vi "CAN Position Control Encoder.vi"() -> ()   [LabVIEW 2014]
doc: "This example shows how to position a motor using CAN Jaguar and a quadrature encoder. For details setting up and understanding CAN Jaguar, see the Can Jaguar Fundamentals tutorial accessable from the LabVIEW Getting Started Window.\n\nTo position the motor, a PID control loop runs on the Jaguar. Notice that the encoder is wired directly to the Jaguar. One advantage of this is that the PID control does not use resources on the roboRIO. One disadvantage is that the PID code cannot be viewed or changed. However, the control can be tuned by changing the PID Parameters.\n\nOn the diagram, notice that in order to apply new PID tuning parameters, the motor must first be disabled, and then enabled afterward. Also notice that since the control loop runs on the Jaguar, the LabVIEW loop delay is set to a slow 100ms. In fact the only reason this loop needs to run is to send a new set position, read the current position, or apply new tuning parameters.\n\nCorrect tuning parameters for a PID controller are dependent on the complete system of the motor and the load. It will be difficult to tune this system if there is no load attached to the motor. While this example is not a PID tutorial, the following information may help in understanding how to tune your PID control system.\n\nP (proportional) depends on the present error, I (integral) on the accumulation of past errors, and D (derivative) is a prediction of future errors, based on the current rate of change. The proportional parameter (P) will reduce the rise time and will reduce, but never eliminate, the steady-state error. The integral parameter (I) will eliminate the steady-state error, but may make the transient response worse. The derivative parameter (D) will increase the stability of the system, reducing the overshoot, and improving the transient response. The effects of each parameter are summarized in a table on the front panel.\n\nThis example expects a USB cable connected from your development PC to the Type B USB Jack (next to the power input) on the roboRIO.\n\nThis example requires the Driver Station to be running with Teleoperated Enabled."
uses:
  <vilib>/Rock Robotics/WPI/CAN/Jaguar/SubVIs/WPI_CANJaguar_PositionReference.ctl
  <vilib>/Rock Robotics/WPI/CAN/TalonSRX/WPI_CANTalonSRX_APIControlMode.ctl
  <vilib>/Rock Robotics/WPI/MotorControl/WPI_MotorControlOpenCANTalonSRX.vi
panel:
  in  "PID Tuning":string[][](table)=[["Parameter", "Rise Time", "Overshoot", "Settling\nTime", "Steady State\nError"], ["P", "decrease", "increase", "small\nchange", "decrease"], ["I", "decrease", "increase", "increase", "eliminate"], ["D", "small\nchange", "decrease", "decrease", "small\nchange"]]
  out "Actual Position (revolutions)":dbl(slide) scale=-10.0..10.0
  in  "D2":dbl=15.0 caption="D"
  in  "I2":dbl=0.005 caption="I"
  in  "P2":dbl=500.0 caption="P"
  in  "apply new PID":bool
  in  "D":dbl=15.0
  in  "I":dbl=0.005
  in  "P":dbl=500.0
  in  "Set Position (revolutions)":dbl(slide) scale=-10.0..10.0
  in  "Device Number":u8=1
  in  "stop":bool
  # "Set these inputs before running."
  # "These can be set while running."
  # "Power\nTerminals"
  # "Motor\nTerminals"
  # "Looking at the RJ12 socket on the Jaguar, standard wire colors are shown for an inserted cable.  CAN only uses pins 3 and 4.\npin 3 (red) = CAN H\npin 4 (green) = CAN L"
  # "To roboRIO CAN terminals"
  # "Terminator plug"
  # "Black Jaguar"
  # "A"
  # "B"
  # "Index"
  # "+5V"
  # "Gnd"
  # "Encoder"
  # "white\nblack\nred\ngreen\nyellow\nblue"
  # "1   2   3   4   5   6"
  # "Runtime Tuning"
  # "PID Parameters"
  # "Initial PID Parameters"
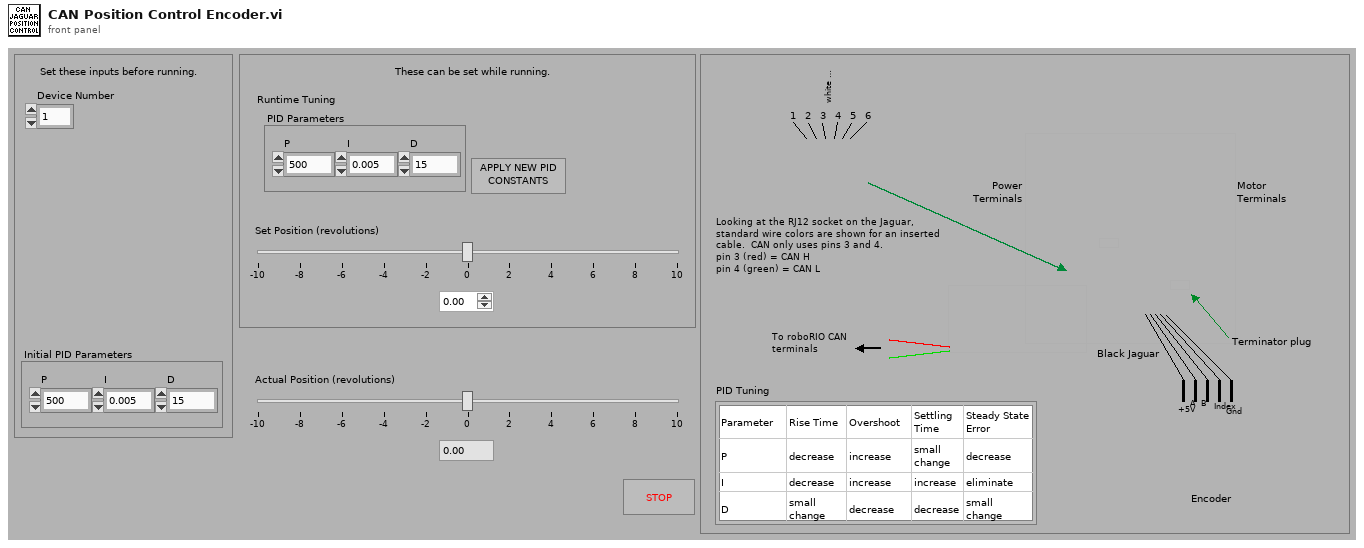
[diagram p1: front panel]
types:
  T1 = typedef "WPI_CANTalonSRX_APIControlMode.ctl" = enum8{"Percent VBus", "Speed", "Position", "Slave", "Unchanged / Invalid"}
  T2 = typedef "WPI_CANJaguar_PositionReference.ctl" = u8
  T3 = typedef "WPI_MotorControlDeviceRef.ctl" = cluster{"DeviceStatus":errorcluster, "Type":T4, "PWM":cluster{"Controller":T5, "PWM Channel":T6, "DeadBand":T7}, "CAN":cluster{"Device Number":u8, "Control Mode":T8, "Semaphore":T9, "Max Vout":dbl, "TalonSRX Control Mode":T1}, "Invert":bool, "TransformRef":T10, "InvTransformRef":T10}
  T4 = typedef "WPI_MotorControlType.ctl" = enum16{"PWM", "CAN", "CANTalonSRX"}
  T5 = typedef "FPGA_TypedefDigitalModule.ctl" = enum16{"Controller 1"}
  T6 = typedef "FPGA_DIOPWMChannel.ctl" = enum8{"PWM 0", "PWM 1", "PWM 2", "PWM 3", "PWM 4", "PWM 5", "PWM 6", "PWM 7", "PWM 8", "PWM 9", "PWM MXP 0", "PWM MXP 1", "PWM MXP 2", "PWM MXP 3", "PWM MXP 4", "PWM MXP 5", "PWM MXP 6", "PWM MXP 7", "PWM MXP 8", "PWM MXP 9", "Invalid"}
  T7 = typedef "WPI_PWMDeadband.ctl" = cluster{"Name":string, "maxPositivePwm":i32, "minPositivePwm":i32, "centerPwm":i32, "maxNegativePwm":i32, "minNegativePwm":i32, "angularRange":u16}
  T8 = typedef "WPI_CANJaguar_ControlMode.ctl" = enum8{"Percent VBus", "Current", "Speed", "Position", "Voltage"}
  T9 = typedef "Semaphore RefNum" = refnum<k1>
  T10 = typedef "WPI_PWMTransform_ConPane.ctl" = refnum<vi>
  T11 = typedef "WPI_CANTalonSRX_GlobalStatus.ctl" = cluster{"Applied Throttle":dbl, "Module Enabled":bool, "CAN Error":errorcluster, "Closed Loop Error":dbl, "Forward Limit Switch Closed":bool, "Reverse Limit Switch Closed":bool, "Sensor Position":dbl, "Sensor Velocity":dbl, "Current":dbl, "Sticky Fault - Over Temp":bool, "Sticky Fault - Under Voltage":bool, "Sticky Fault - Forward Limit":bool, "Sticky Fault - Reverse Limit":bool, "Sticky Fault - Forward Soft Limit":bool, "Sticky Fault - Reverse Soft Limit":bool, "Brake is Enabled":bool, "Encoder Position":dbl, "Encoder Velocity":dbl, "Encoder Index Count":dbl, "Encoder A Pin State":bool, "Encoder B Pin State":bool, "Encoder Index Pin State":bool, "Analog In":dbl, "Analog In Velocity":dbl, "Temperature (C)":dbl, "Battery Voltage":dbl}
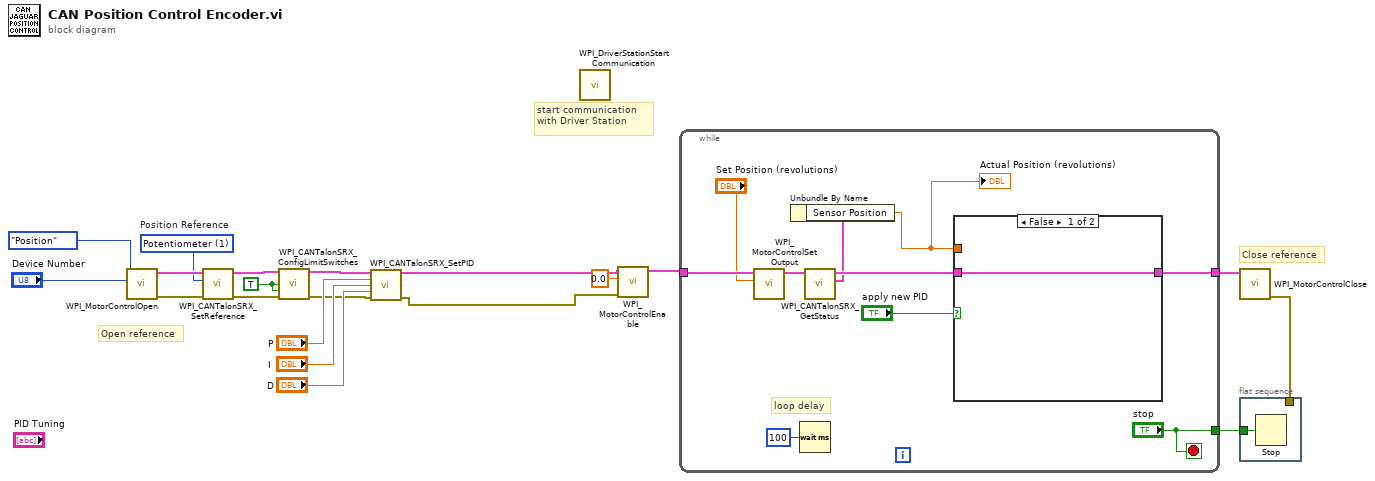
[diagram p0: block diagram]
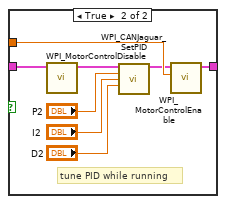
[diagram p2: hidden frame]
diagram:
  w8 = TRUE ("Forward Limit Switch Normally Open")
  w16 = T2 1 items=["Quad Encoder"=0, "Potentiometer"=1, "None"=255]  # Position Reference
  # "Open reference"
  # "start communication with Driver Station"
  # "Close reference"
  n1 = call-poly <vilib>:"WPI_MotorControlOpen.vi"("Device Number"="Device Number", "Control Mode"=WPI_CANTalonSRX_APIControlMode."Position") -> ("error out"=w1:errorcluster, "MotorControlDeviceRef"=w19:T3)  [unwired: 5 in, 3 out]
  n2 = call <vilib>:"WPI_CANTalonSRX_SetReference.vi"("error in (no error)"=w1, "Feedback Reference"=w16, "CAN Talon SRX Ref"=w19) -> ("error out"=w4:errorcluster, "CAN Talon SRX Ref Out"=w18:T3)  [unwired: 7 in]
  n3 = call <vilib>:"WPI_CANTalonSRX_ConfigLimitSwitches.vi"("CAN Talon SRX Ref"=w18, "Forward Limit Switch Normally Open"=w8, "Reverse Limit Switch Normally Open"=w8, "error in (no error)"=w4) -> ("CAN Talon SRX Ref Out"=w17:T3, "error out"=w3:errorcluster)  [unwired: 10 in]
  n4 = call <vilib>:"WPI_CANTalonSRX_SetPID.vi"("CAN Talon SRX Ref"=w17, "P"="P", "I"="I", "D"="D", "error in (no error)"=w3) -> ("CAN Talon SRX Ref Out"=w6:T3, "error out"=w2:errorcluster)  [unwired: 9 in]
  n5 = call <vilib>:"WPI_DriverStationStart Communication.vi"() -> ()  [unwired: 2 in, 10 out]
  n6 = call <vilib>:"WPI_MotorControlEnable.vi"("error in (no error)"=w2, "Encoder Initial Position"=0.0, "CAN Jaguar Ref"=w6) -> ("CAN Jaguar Ref Out"=w7:T3)  [unwired: 7 in, 1 out]
  n7 = while {
    tunnel: ["stop"] -> w11
    tunnel: w7 -> [w28]
    tunnel: [w25] -> w15
    stop <- "stop" stop-if-true
    # "loop delay"
    n8 = call <vilib>:"WPI_MotorControlSetOutput.vi"("Output"="Set Position (revolutions)", "MotorControlDevRef"=w28) -> ("MotorControlDevRef"=w27:T3)  [unwired: 7 in, 2 out]
    n9 = Wait (ms)(milliseconds to wait=u32 100) -> ()  [unwired: 1 out]
    n10 = call <vilib>:"WPI_CANTalonSRX_GetStatus.vi"("CAN Talon SRX Ref"=w27) -> ("Talon SRX Status"=w22:T11, "CAN Talon SRX Ref Out"=w26:T3)  [unwired: 8 in, 1 out]
    n11 = Unbundle By Name(w22) -> ("Sensor Position"=w21:dbl)
    "Actual Position (revolutions)" <- w21
    n12 = case shown="False" "apply new PID" {
      tunnel: w26 -> [w31 w36]
      tunnel: w21 -> [_ w39]
      tunnel: [w31 w37] -> w25
      frame False {
      }
      frame True {
        # "tune PID while running"
        n13 = call <vilib>:"WPI_MotorControlDisable.vi"("MotorControlDevRef"=w36) -> ("MotorControlDevRef"=w35:T3)  [unwired: 9 in, 1 out]
        n14 = call <vilib>:"WPI_CANJaguar_SetPID.vi"("CAN Jaguar Ref"=w35, "P"="P2", "I"="I2", "D"="D2") -> ("CAN Jaguar Ref Out"=w38:T3)  [unwired: 10 in, 1 out]
        n15 = call <vilib>:"WPI_MotorControlEnable.vi"("Encoder Initial Position"=w39, "CAN Jaguar Ref"=w38) -> ("CAN Jaguar Ref Out"=w37:T3)  [unwired: 8 in, 1 out]
      }
    }
  }
  n16 = call <vilib>:"WPI_MotorControlClose.vi"("MotorControlDevRef"=w15) -> ("error out"=w10:errorcluster)  [unwired: 10 in]
  n17 = flat-sequence {
    tunnel: w11 -> [w40]
    tunnel: w10 -> [_]
    frame #0 {
      n18 = Stop(stop? (T)=w40) -> ()
    }
  }
